vi "Reset Measurements (Peak Only).vi"(0 "VISA resource name":refnum<visa-resource-name>, 11 "error in (no error)":errorcluster) -> (4 "VISA resource name out":refnum<visa-resource-name>, 15 "error out":errorcluster)   [LabVIEW 2020, in "NH Research Regenerative Test Series.lvlib"]
doc: "Resets all accumulated peak measurements:\n\nVoltageNegativePeak, VoltagePositivePeak, CurrentNegativePeak, CurrentPositivePeak, PowerNegativePeak, PowerPositivePeak."
uses:
  NH Research Regenerative Test Series.lvlib
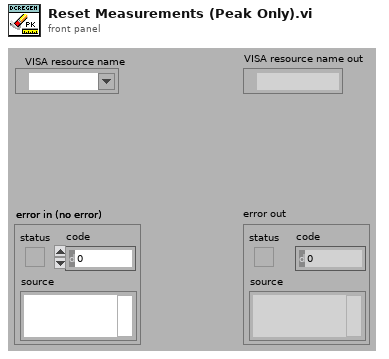
[diagram p1: front panel]
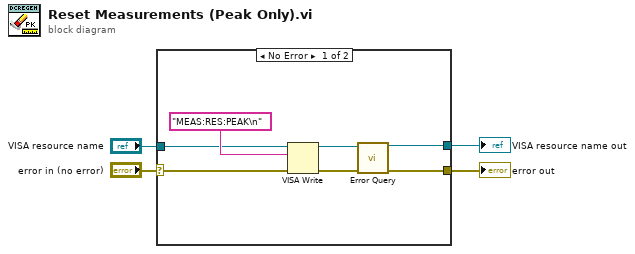
[diagram p0: block diagram]
diagram:
  n1 = case shown="No Error" "error in (no error)" {
    selector: "error in (no error)" -> [w7 w12]
    tunnel: "VISA resource name" -> [w10 w13]
    tunnel: [w9 w13] -> w3
    tunnel: [w8 w12] -> w2
    frame No Error {
      n2 = VISA Write(VISA resource name=w10, write buffer="MEAS:RES:PEAK\n" ("Command to Send (empty)"), error in (no error)=w7) -> (VISA resource name out=w6:refnum<visa-resource-name>, error out=w5:errorcluster)  [unwired: 1 out]
      n3 = call "Error Query.vi"("VISA resource name"=w6, "error in (no error)"=w5) -> ("VISA resource name out"=w9:refnum<visa-resource-name>, "error out"=w8:errorcluster)  [unwired: 10 in, 2 out]
    }
    frame Error {
    }
  }
  "error out" <- w2
  "VISA resource name out" <- w3
